vi "sub parse frame w.vi"(8 "error in (no error)":errorcluster, 11 "<w> String":string="   <bp x 56.88426948876875 y 39.15890324252262 bp>") -> (0 "error out":errorcluster, 3 "w data":T1)   [LabVIEW 2018, in "Data Parser.lvclass"]
uses:
  Data Parser.lvclass
  frame w data.ctl
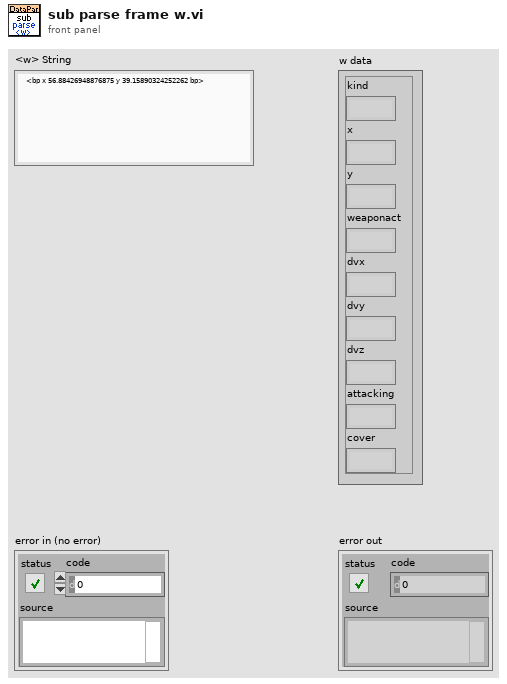
[diagram p1: front panel]
types:
  T1 = typedef "Data Parser.lvclass/frame w data.ctl" = cluster{"kind":string, "x":string, "y":string, "weaponact":string, "dvx":string, "dvy":string, "dvz":string, "attacking":string, "cover":string}
  T2 = cluster{"[0]":string, "[1]":string, "[2]":string, "[3]":string, "[4]":string, "[5]":string, "[6]":string, "[7]":string, "[8]":string}
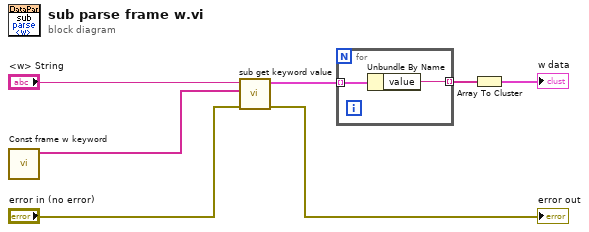
[diagram p0: block diagram]
diagram:
  n1 = call "Const frame w keyword.vi"() -> ("Const frame w keyword"=w1:string[])  [unwired: 11 in]
  n2 = call "sub get keyword value.vi"("error in"="error in (no error)", "keyword"=w1, "string"="<w> String") -> ("error out"=→"error out":errorcluster, "matched pairs (all)"=w4:cluster{"keyword":string, "value":string}[])  [unwired: 5 in, 2 out]
  n3 = for {
    tunnel: w4 -> [w9] mode=indexing
    tunnel: [w8] -> w3 mode=indexing
    n4 = Unbundle By Name(w9) -> ("value"=w8:string)
  }
  n5 = Array To Cluster(array=w3) -> (cluster=→"w data":T2)
